vi "SynchiIO.PXI4461.API_TEMPLATE.vi"(8 "error in (no error)":errorcluster, 10 "myData":string, 11 "SynchiIO.PXI4461":refnum<class "SynchiIO.PXI4461.lvclass">) -> (0 "error out":errorcluster, 2 "Data out":string, 3 "SynchiIO.PXI4461 out":refnum<class "SynchiIO.PXI4461.lvclass">)   [LabVIEW 2016, in "SynchiIO.PXI4461.lvclass"]
doc: "---------------------------------------------------------------\nJKI State Machine Objects™\nhttp://jki.net/state-machine-objects/\nCopyright (C) 2005-2015, JKI <info@jki.net>\nALL RIGHTS RESERVEDJKI State Machine Objects (SMO) 1.0.0.5\nJKI - JKI\nCopyright (c) 2016, JKI"
uses:
  SynchiIO.PXI4461.lvclass
  Typedefs/API Inputs--Cluster.ctl
panel:
  # "For instructions on how to use the JKI State Machine Objects, examples and video tutorials, visit:\nhttp://jki.net/state-machine-objects/\n\nJKI State Machine Objects™\nhttp://jki.net/state-machine-objects/\nCopyright (C) 2005-2015, JKI <info@jki.net>\nALL RIGHTS RESERVED"
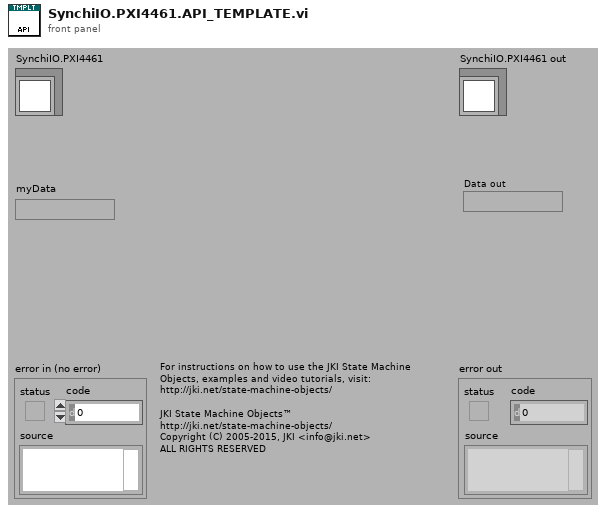
[diagram p1: front panel]
types:
  T1 = typedef "SynchiIO.PXI4461.lvclass/API Inputs--Cluster.ctl" = cluster{"Data":string}
  T2 = typedef "SynchiIO.PXI4461.lvclass/ProtectedEvents--Cluster.ctl" = cluster{"API_Template":refnum<user-event>}
  T3 = typedef "SynchiIO.PXI4461.lvclass/PrivateData--Ref.ctl" = refnum<data-value>
  T4 = typedef "SynchiIO.PXI4461.lvclass/PrivateData--Cluster.ctl" = cluster{"Configuration":T5, "Public Events":T6, "Protected Events":T2, "Data":string}
  T5 = typedef "SynchiIO.PXI4461.lvclass/Configuration--Cluster.ctl" = cluster{"Suffix":string}
  T6 = typedef "SynchiIO.PXI4461.lvclass/PublicEvents--Cluster.ctl" = cluster{"Data Changed":refnum<user-event>}
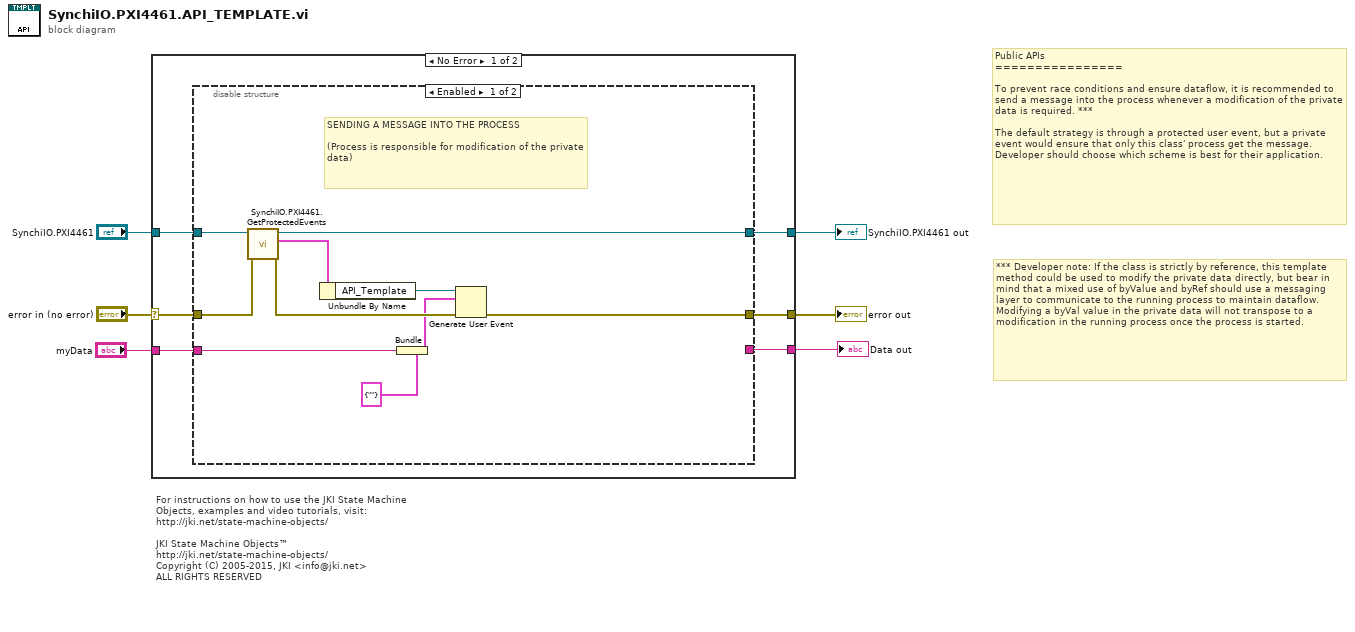
[diagram p0: block diagram]
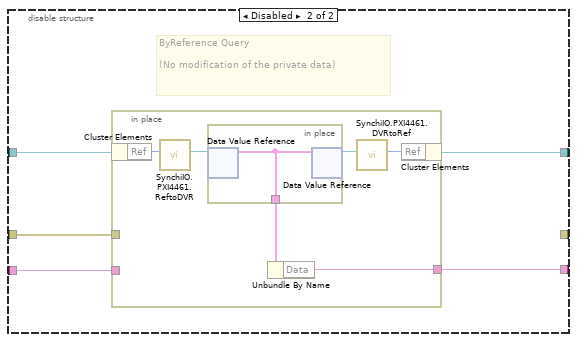
[diagram p2: hidden frame]
diagram:
  # "*** Developer note: If the class is strictly by reference, this template method could be used to modify the private data directly, but bear in mind that a mixed use of byValue and byRef should use a messaging layer to communicate to the running process to maintain dataflow. Modifying a byVal value in the private data will not transpose to a modification in the running process once the process is started."
  # "Public APIs\n================\n\nTo prevent race conditions and ensure dataflow, it is recommended to send a message into the process whenever a modification of the private data is required. ***\n\nThe default strategy is through a protected user event, but a private event would ensure that only this class' process get the message. Developer should choose which scheme is best for their application."
  # "For instructions on how to use the JKI State Machine Objects, examples and video tutorials, visit:\nhttp://jki.net/state-machine-objects/\n\nJKI State Machine Objects™\nhttp://jki.net/state-machine-objects/\nCopyright (C) 2005-2015, JKI <info@jki.net>\nALL RIGHTS RESERVED"
  n1 = case shown="No Error" "error in (no error)" {
    selector: "error in (no error)" -> [w11 w35]
    tunnel: "SynchiIO.PXI4461" -> [w8 w36]
    tunnel: [w10 w35] -> w5
    tunnel: [w9 w36] -> w4
    tunnel: "myData" -> [w12 _]
    tunnel: [w7 _] -> w1
    frame No Error {
      n2 = disable-structure shown="Enabled" {
        disable-tunnel: w12 -> [w21 w24]
        disable-tunnel: w11 -> [w20 w25]
        disable-tunnel: [w15 _] -> w10
        disable-tunnel: [w14 w26] -> w9
        disable-tunnel: w8 -> [w13 w27]
        disable-tunnel: [_ w23] -> w7
        frame Enabled {
          # "SENDING A MESSAGE INTO THE PROCESS\n\n(Process is responsible for modification of the private data)"
          n3 = call "SynchiIO.PXI4461.GetProtectedEvents.vi"("error in (no error)"=w20, "SynchiIO.PXI4461"=w13) -> ("error out"=w18:errorcluster, "Protected Events"=w19:T2, "SynchiIO.PXI4461 out"=w14:refnum<class "SynchiIO.PXI4461.lvclass">)  [unwired: 7 in]
          n4 = Unbundle By Name(w19) -> ("API_Template"=w22:refnum<user-event>)
          n5 = Bundle(cluster=T1 {"Data"=""} ("event data"), "Data"=w21) -> (w16:T1)
          n6 = Generate User Event(user event=w22, event data cluster=w16, error in=w18) -> (error out=w15:errorcluster)  [unwired: 1 in, 1 out]
        }
        frame Disabled {
          # "ByReference Query\n\n(No modification of the private data)"
          n7 = in-place {
            in-place-border: w25 -> [_]
            in-place-border: w24 -> [_]
            in-place-border: [w28] -> w23
            n8 = in-place-cluster #1(w27) -> ("Ref"=w32:u32)
            n9 = call "SynchiIO.PXI4461.ReftoDVR.vi"("Ref"=w32) -> ("Ref"=w33:T3)  [unwired: 10 in]
            n10 = in-place {
              in-place-border: [w34] -> w29
              n11 = in-place-dvr #2(w33) -> (w34:T4)  [unwired: 1 out]
              n12 = in-place-dvr #2(w34) -> (w31:T3)  [unwired: 1 out]
            }
            n13 = Unbundle By Name(w29) -> ("Data"=w28:string)
            n14 = call "SynchiIO.PXI4461.DVRtoRef.vi"("Ref"=w31) -> ("Ref"=w30:u32)  [unwired: 10 in]
            n15 = in-place-cluster #1("Ref"=w30) -> (w26:refnum<class "SynchiIO.PXI4461.lvclass">)
          }
        }
      }
    }
    frame Error {
    }
  }
  "error out" <- w5
  "SynchiIO.PXI4461 out" <- w4
  "Data out" <- w1
